vi "Initialize With Options.vi"(7 "option string":string, 8 "error in (no error)":errorcluster {"code" format="%.0x"}, 9 "reset device (Off)":bool, 10 "id query (Off)":bool, 11 "resource string":string caption="resource name") -> (0 "error out":errorcluster {"code" format="%.0x"}, 3 "instrument handle out":refnum<k15>)   [LabVIEW 2009, in "Keysight XSAn.lvlib"]
doc: "Opens the I/O session to the instrument. Driver methods and properties that access the instrument are only accessible after Initialize is called. Initialize optionally performs a Reset and queries the instrument to validate the instrument model.\n\nSupported Models: All supported"
uses:
  <instrlib>/Keysight XSAn/Keysight XSAn.lvlib
  AgXSAn.dll
panel:
  # "© Keysight Technologies 2015-2021"
  # "© 2000-2008 National Instruments.  All Rights Reserved."
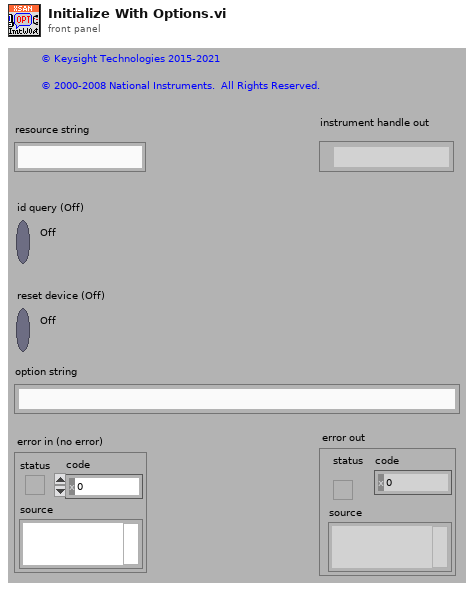
[diagram p1: front panel]
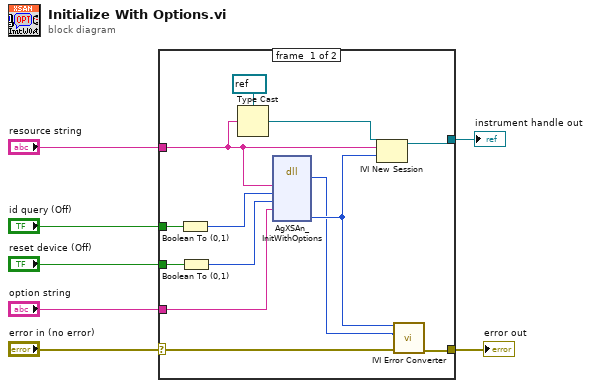
[diagram p0: block diagram]
diagram:
  n1 = case shown="No Error" "error in (no error)" {
    selector: "error in (no error)" -> [w8 w22]
    tunnel: [w11 w22] -> w1
    tunnel: "resource string" -> [w14 w21]
    tunnel: [w18 w21] -> w2
    tunnel: "id query (Off)" -> [w17 _]
    tunnel: "reset device (Off)" -> [w16 _]
    tunnel: "option string" -> [w15 _]
    frame #0 {
      n2 = Boolean To (0,1)(Boolean=w17) -> (0, 1=w20:i16)
      n3 = Boolean To (0,1)(Boolean=w16) -> (0, 1=w19:i16)
      n4 = Type Cast(type=refnum<k15> refnum ("instrument handle out 2"), x=w14) -> (*(type *) &x=w13:refnum<k15>)
      n5 = dll-call lib="AgXSAn**.dll" fn="AgXSAn_InitWithOptions" ("LabVIEW:Ivi_InitWithOptionsAndGetError")("resourceDescriptor"=w14, "idQuery"=w20, "reset"=w19, "optionString"=w15) -> ("return type"=w9:i32, "session"=w10:i32)  [unwired: 6 in, 4 out]
      n6 = IVI New Session(9:w10, 10:w14, 11:w13) -> (3:w18:refnum<k15>)
      n7 = call <instrlib>:"IVI Error Converter.vi"("error in (no error)"=w8, "IVI error code (0)"=w9, "instrument handle"=w10) -> ("error out"=w11:errorcluster)  [unwired: 7 in, 1 out]
    }
    frame #1 {
    }
  }
  "error out" <- w1
  "instrument handle out" <- w2
